vi "Globals.vi"() -> ()   [LabVIEW 2017, in "nifxpmath_Convert.xnode"]
uses:
  <vilib>/rvi/FXPMathLib/FxpConvert/XNode/nifxpmath_Convert.xnode
panel:
  out "SMALLICON w/ 4WIRE":picture
  in  "TERM Y NAME":string="y"
  in  "TERM X NAME":string="x"
  in  "TERM OVFL ID":string="TERM_OVFL"
  in  "TERM Y ID":string="TERM_Y"
  in  "TERM X ID":string="TERM_X"
  out "SMALLICON":picture
  out "NORMALBANNER":picture
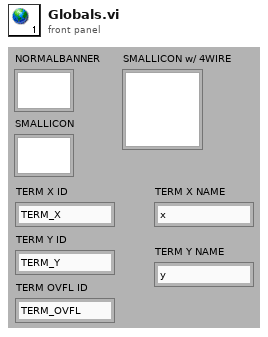
[diagram p1: front panel]
diagram:
